vi "Launch Nested.vi"(8 "error in (no error)":errorcluster, 11 "Main GUI in":refnum<class "Main GUI.lvclass">) -> (0 "error out":errorcluster, 3 "Main GUI out":refnum<class "Main GUI.lvclass">)   [LabVIEW 2019, in "Main GUI.lvlib" / "Main GUI.lvclass"]
uses:
  Main GUI.lvclass
  C:/Program Files (x86)/National Instruments/LabVIEW 2019/vi.lib/ActorFramework/Actor/Actor.lvclass
  Nested/Nested/Nested.lvclass
  <vilib>/ActorFramework/Actor/Actor.lvclass
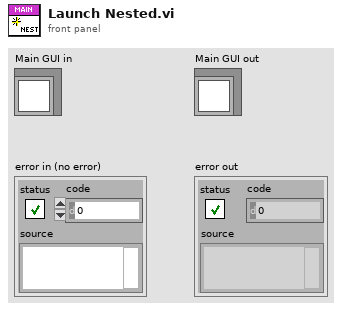
[diagram p1: front panel]
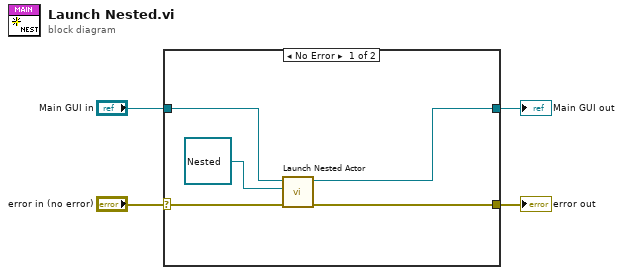
[diagram p0: block diagram]
diagram:
  n1 = case shown="No Error" "error in (no error)" {
    selector: "error in (no error)" -> [w9 w11]
    tunnel: [w8 w11] -> w3
    tunnel: [w5 w10] -> w1
    tunnel: "Main GUI in" -> [w7 w10]
    frame No Error {
      n2 = call <vilib>:"Launch Nested Actor.vi"("error in (no error)"=w9, "Nested Actor"=refnum<class "Nested.lvclass"> refnum ("Pop Up.lvlib:Pop Up.lvclass"), "Caller Actor in"=w7) -> ("error out"=w8:errorcluster, "Caller Actor out"=w5:refnum<class "Main GUI.lvclass">)  [unwired: 6 in, 1 out]
    }
    frame Error {
    }
  }
  "error out" <- w3
  "Main GUI out" <- w1
